vi "Alt_Facade.vi"(0 "Data In":T7, 2 "Display State In":T5, 3 "Container State":T6) -> (6 "Data Out":T7, 7 "Display State Out":T5, 8 "Action":T4)   [LabVIEW 2013, in "Alt.xctl"]
uses:
  Alt.xctl
  <vilib>/_xctls/Action.ctl
  <vilib>/_xctls/XControlSupport.lvlib
  <vilib>/_xctls/Container State.ctl
  Alt_Data.ctl
  Alt_State.ctl
  Type Defs/Alt Digit 100 New.ctl
  Type Defs/Alt Control.ctl
  Type Defs/Current Alt Set.ctl
panel:
  out "CURRENT ALT SET":T1 caption="Current Set Point" format="%#.0f"
  in  "Confirm Now":bool
  in  "ALT SET 2":T2 {"Alt Digit 100" min=0 max=9 step=1; "Alt Digit 100" min=0 max=9 step=1; "Alt Digit 100" min=0 max=9 step=1; "Alt Digit 100" min=0 max=9 step=1; "Alt Digit 100" min=0 max=9 step=1}
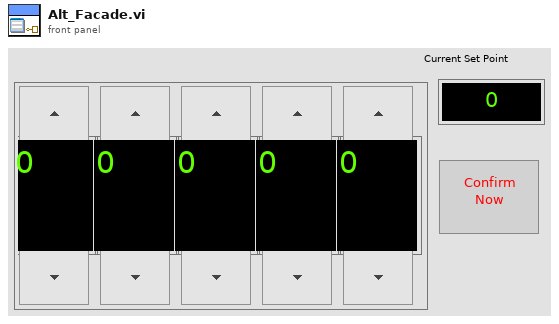
[diagram p1: front panel]
types:
  T1 = typedef "Current Alt Set.ctl" = i32
  T2 = typedef "Alt Control.ctl" = cluster{"Alt Digit 100":T3, "Alt Digit 100":T3, "Alt Digit 100":T3, "Alt Digit 100":T3, "Alt Digit 100":T3}
  T3 = typedef "Alt Digit 100 New.ctl" = i8
  T4 = typedef "XControlSupport.lvlib/Action.ctl" = cluster{"Data Changed?":bool, "State Changed?":bool, "Action Name":string}
  T5 = typedef "Alt.xctl/Alt_State.ctl" = cluster{"Numeric":dbl}
  T6 = typedef "XControlSupport.lvlib/Container State.ctl" = cluster{"Indicator?":bool, "Run Mode?":bool, " Refnum":refnum<vi>}
  T7 = typedef "Alt.xctl/Alt_Data.ctl" = i32
  T8 = cluster{"[0]":i8, "[1]":i8, "[2]":i8, "[3]":i8, "[4]":i8}
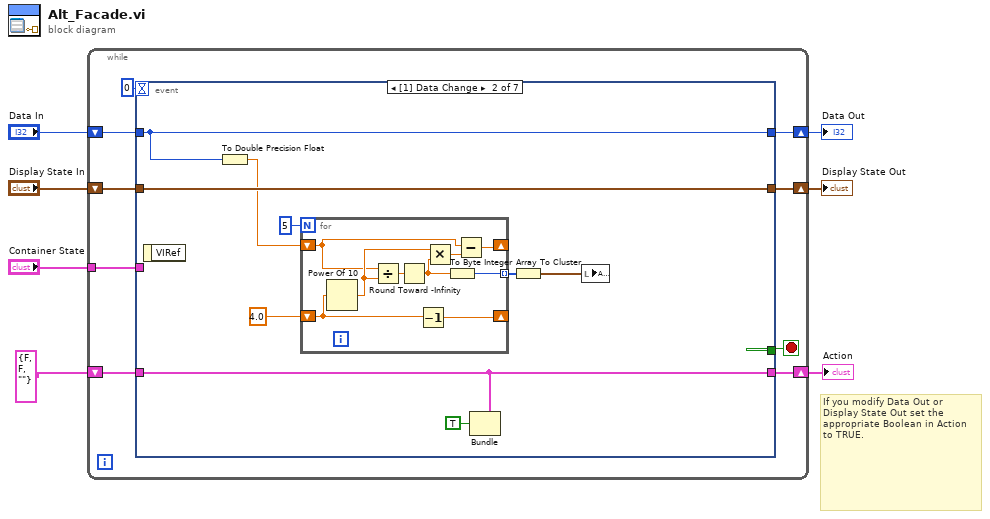
[diagram p0: block diagram]
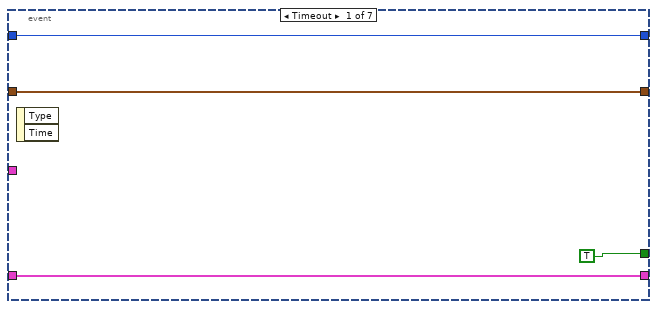
[diagram p2: hidden frame]
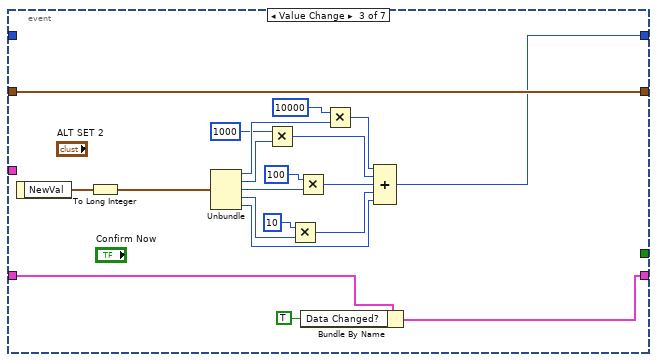
[diagram p3: hidden frame]
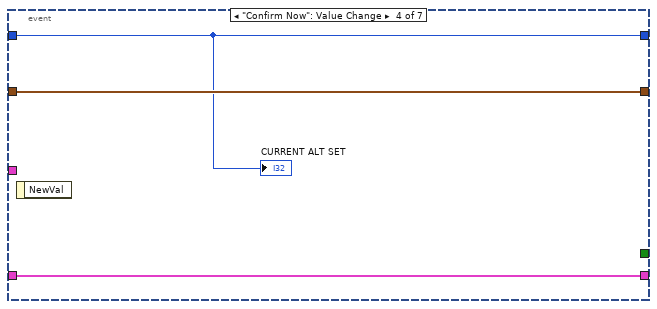
[diagram p4: hidden frame]
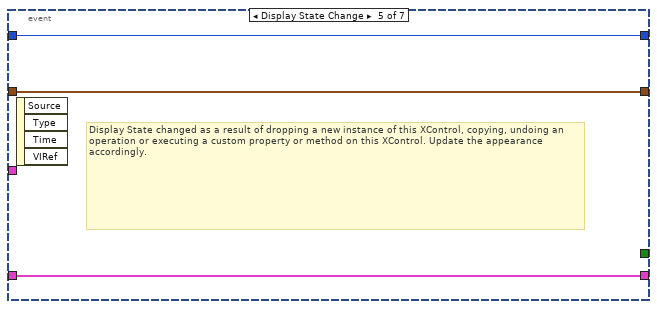
[diagram p5: hidden frame]
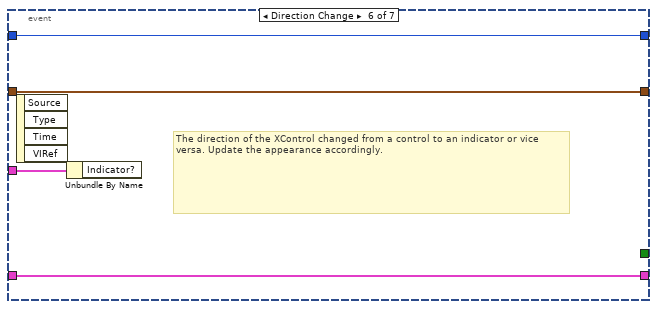
[diagram p6: hidden frame]
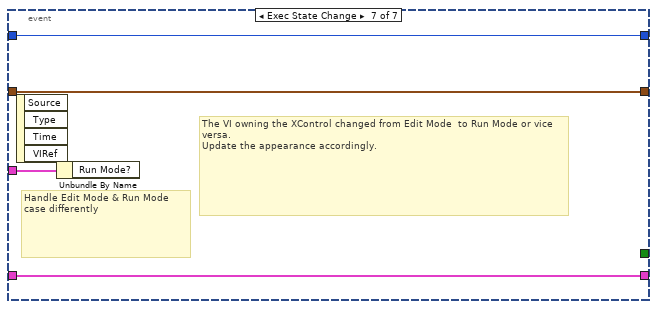
[diagram p7: hidden frame]
diagram:
  # "If you modify Data Out or\nDisplay State Out set the\nappropriate Boolean in Action\nto TRUE."
  n1 = while {
    shift-right: [w15] -> w4
    shift-left: "Display State In" -> [w16]
    tunnel: "Container State" -> [w12]
    shift-right: [w10] -> w7
    shift-left: "Data In" -> [w11]
    shift-right: [w8] -> w2
    shift-left: T4 {"Data Changed?"=FALSE, "State Changed?"=FALSE, "Action Name"=""} ("Action") -> [w9]
    stop <- w14 stop-if-true
    n2 = event shown="[1] Data Change" {
      selector: _ -> [_ _ _ _ _ _ _]
      dyn-events: _ -> [_ _ _ _ _ _ _]
      timeout: 0 -> [_ _ _ _ _ _ _]
      tunnel: w16 -> [w18 w29 w58 w61 w64 w67 w71]
      tunnel: [w18 w29 w58 w61 w64 w67 w71] -> w15
      tunnel: [TRUE _ _ _ _ _ _] -> w14
      tunnel: w12 -> [_ _ _ _ _ w68 w72]
      tunnel: w11 -> [w17 w25 _ w59 w63 w66 w70]
      tunnel: [w17 w25 w44 w59 w63 w66 w70] -> w10
      tunnel: [w19 w22 w39 w60 w62 w65 w69] -> w8
      tunnel: w9 -> [w19 w22 w41 w60 w62 w65 w69]
      event Timeout {
        n3 = event-data() -> ()  [unwired: 1 in, 2 out]
      }
      event Data Change {
        n4 = event-data() -> ()  [unwired: 1 in, 1 out]
        n5 = To Double Precision Float(number=w25) -> (double precision float=w28:dbl)
        n6 = for {
          N: 5 -> [_]
          shift-right: [w30] -> _
          shift-left: w28 -> [w31]
          tunnel: [w37] -> w24 mode=indexing
          shift-right: [w36] -> _
          shift-left: 4.0 -> [w35]
          n7 = Power Of 10(x=w35) -> (10^x=w33:dbl)
          n8 = Divide(x=w31, y=w33) -> (x/y=w38:dbl)
          n9 = Round Toward -Infinity(1:w38) -> (0:w34:dbl)
          n10 = Decrement(x=w35) -> (x-1=w36:dbl)
          n11 = Multiply(x=w33, y=w34) -> (x*y=w32:dbl)
          n12 = To Byte Integer(number=w34) -> (8bit integer=w37:i8)
          n13 = Subtract(x=w31, y=w32) -> (x-y=w30:dbl)
        }
        n14 = Bundle(cluster=w22, "State Changed?"=TRUE) -> ()  [unwired: 2 in, 1 out]
        n15 = Array To Cluster(array=w24) -> (cluster=w23:T8)
        n16 = local write item#-1(w23) -> ()
      }
      event Value Change {
        n17 = event-data() -> ("NewVal"=w43:T2)  [unwired: 1 in]
        n18 = To Long Integer(number=w43) -> (32bit integer=w42:cluster{i32, i32, i32, i32, i32})
        n19 = Unbundle(w42) -> (w57:i32, w52:i32, w51:i32, w50:i32, w45:i32)
        n20 = Multiply(x=1000, y=w52) -> (x*y=w48:i32)
        n21 = Multiply(x=10, y=w50) -> (x*y=w46:i32)
        n22 = Multiply(x=100, y=w51) -> (x*y=w47:i32)
        n23 = Bundle By Name(cluster=w41, "Data Changed?"=TRUE) -> (w39:T4)
        n24 = Multiply(x=10000, y=w57) -> (x*y=w49:i32)
        n25 = Compound Arithmetic op=ADD(w49, w48, w47, w46, w45) -> (w44:i32)
      }
      event "Confirm Now": Value Change {
        n26 = event-data() -> ()  [unwired: 1 in, 1 out]
        "CURRENT ALT SET" <- w59
      }
      event Display State Change {
        # "Display State changed as a result of dropping a new instance of this XControl, copying, undoing an operation or executing a custom property or method on this XControl. Update the appearance accordingly."
        n27 = event-data() -> ()  [unwired: 1 in, 4 out]
      }
      event Direction Change {
        # "The direction of the XControl changed from a control to an indicator or vice versa. Update the appearance accordingly."
        n28 = event-data() -> ()  [unwired: 1 in, 4 out]
        n29 = Unbundle By Name(w68) -> ()  [unwired: 1 out]
      }
      event Exec State Change {
        # "The VI owning the XControl changed from Edit Mode  to Run Mode or vice versa.\nUpdate the appearance accordingly."
        # "Handle Edit Mode & Run Mode\ncase differently"
        n30 = event-data() -> ()  [unwired: 1 in, 4 out]
        n31 = Unbundle By Name(w72) -> ()  [unwired: 1 out]
      }
    }
  }
  "Display State Out" <- w4
  "Data Out" <- w7
  "Action" <- w2
